vi "FTW-Request-Body.vi"(0 "FTW Request":refnum<class "FTW-Request.lvclass">, 11 "error in":errorcluster) -> (4 "FTW Request out":refnum<class "FTW-Request.lvclass">, 6 "Request Body":string, 15 "error out":errorcluster)   [LabVIEW 2014, in "FTW-Request.lvclass"]
uses:
  FTW-Request.lvclass
  FTW-Request.lvclass/FTW-Request.ctl
  json/FTW-JSON.lvclass
panel:
  # "Inputs"
  # "Outputs"
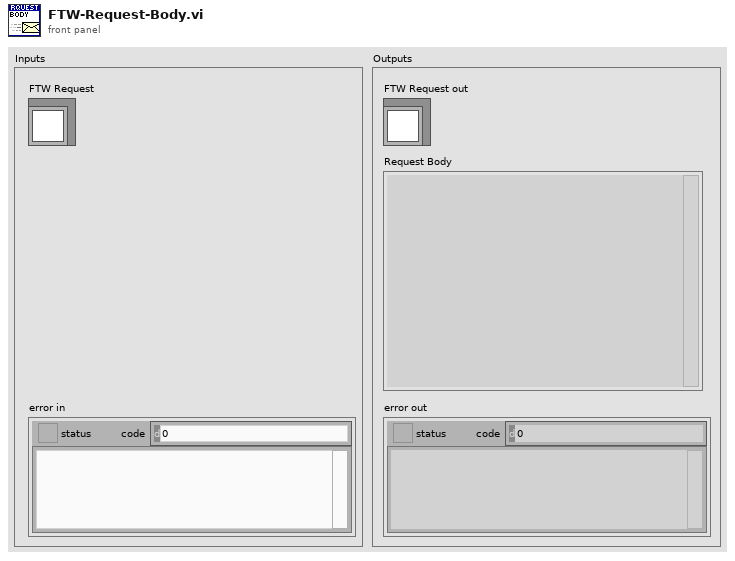
[diagram p1: front panel]
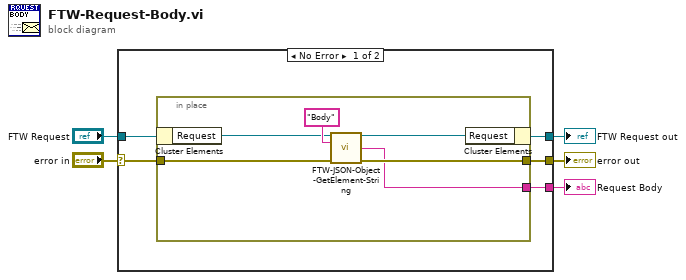
[diagram p0: block diagram]
diagram:
  n1 = case shown="No Error" "error in" {
    selector: "error in" -> [w8 w17]
    tunnel: [w7 w17] -> w2
    tunnel: [w9 w18] -> w3
    tunnel: "FTW Request" -> [w10 w18]
    tunnel: [w6 _] -> w1
    frame No Error {
      n2 = in-place {
        in-place-border: w8 -> [w12]
        in-place-border: [w14] -> w7
        in-place-border: [w11] -> w6
        n3 = in-place-cluster #1(w10) -> ("Request"=w13:refnum<class "FTW-JSON.lvclass">)
        n4 = call "FTW-JSON-Object-GetElement-String.vi"("JSON Object"=w13, "Key"="Body", "error in"=w12) -> ("JSON Object out"=w16:refnum<class "FTW-JSON.lvclass">, "Value"=w11:string, "error out"=w14:errorcluster)  [unwired: 9 in, 1 out]
        n5 = in-place-cluster #1("Request"=w16) -> (w9:refnum<class "FTW-Request.lvclass">)
      }
    }
    frame Error {
    }
  }
  "error out" <- w2
  "Request Body" <- w1
  "FTW Request out" <- w3
